vi "Harness_Run All Jitter Tests Reentrancy_Pretest.vi"(10 "Results FilePath":path, 11 "Jitter Test Folder":path) -> ()   [LabVIEW 2009]
panel:
  out "error out":errorcluster
  in  "Run in UI?":bool
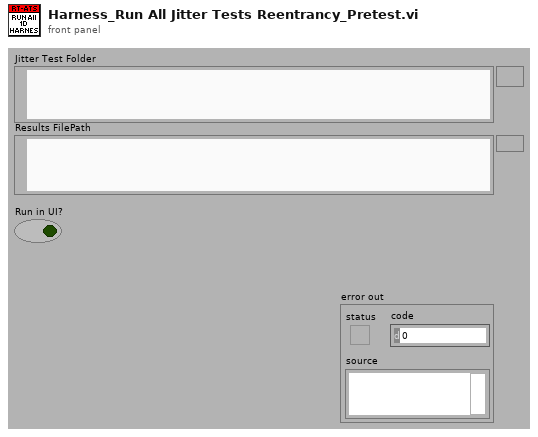
[diagram p1: front panel]
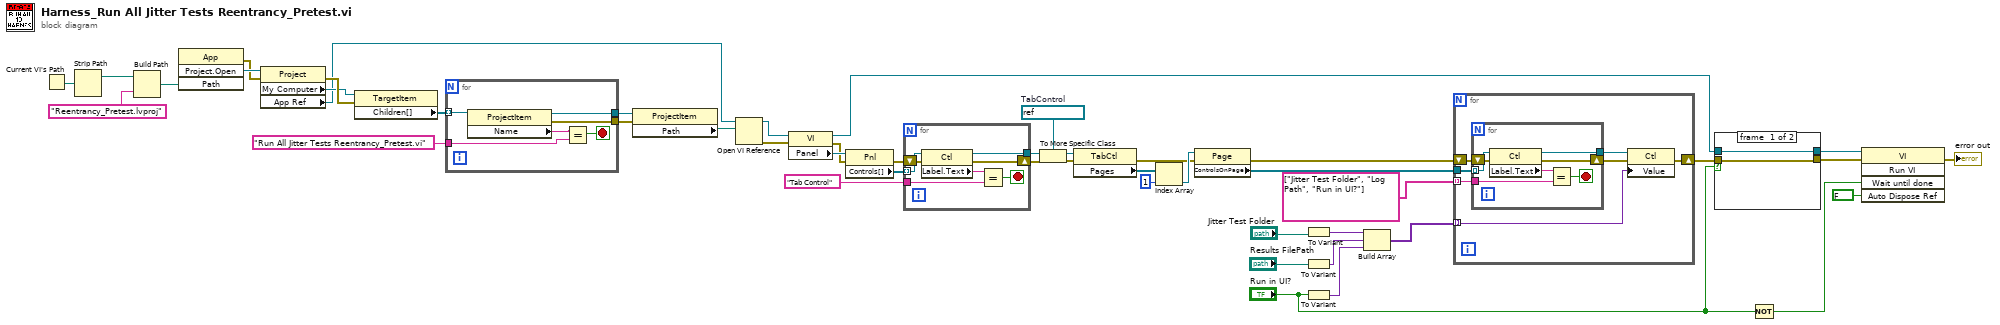
[diagram p0: block diagram]
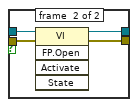
[diagram p2: hidden frame]
diagram:
  w9 = refnum<vi> refnum  # TabControl
  n1 = Current VI's Path() -> (path=w47:path)
  n2 = Strip Path(path=w47) -> (stripped path=w46:path)  [unwired: 1 out]
  n3 = Build Path(base path=w46, name or relative path="Reentrancy_Pretest.lvproj") -> (appended path=w44:path)
  n4 = invoke class="App" method="Project.Open"("Path"=w44) -> (error out=w42:errorcluster, "Project:Open"=w43:refnum<vi>)  [unwired: 3 in, 2 out]
  n5 = property class="Project"(reference=w43, error in=w42) -> (error out=w41:errorcluster, "My Computer"=w35:refnum<vi>, "App Ref"=w34:refnum<vi>)  [unwired: 1 out]
  n6 = property class="TargetItem"(reference=w35, error in=w41) -> ("Children[]"=w40:refnum<vi>[])  [unwired: 2 out]
  n7 = for {
    tunnel: w40 -> [w53] mode=indexing
    tunnel: "Run All Jitter Tests Reentrancy_Pretest.vi" ("name or relative path") -> [w51]
    tunnel: [w49] -> w38
    tunnel: [w48] -> w37
    stop <- w50 stop-if-true
    n8 = property class="ProjectItem"(reference=w53) -> (reference out=w49:refnum<vi>, error out=w48:errorcluster, "Name"=w52:string)  [unwired: 1 in]
    n9 = Equal?(x=w52, y=w51) -> (x = y?=w50:bool)
  }
  n10 = property class="ProjectItem"(reference=w38, error in=w37) -> ("Path"=w36:path)  [unwired: 2 out]
  n11 = Open VI Reference(application reference (local)=w34, vi path=w36) -> (vi reference=w32:refnum<vi>, error out=w33:errorcluster)  [unwired: 4 in]
  n12 = property class="VI"(reference=w32, error in=w33) -> (reference out=w21:refnum<vi>, error out=w30:errorcluster, "Panel"=w31:refnum<vi>)
  n13 = property class="Pnl"(reference=w31, error in=w30) -> (error out=w14:errorcluster, "Controls[]"=w12:refnum<vi>[])  [unwired: 1 out]
  n14 = for {
    tunnel: w12 -> [w59] mode=indexing
    tunnel: "Tab Control" -> [w57]
    tunnel: [w55] -> w11
    shift-right: [w54] -> w10
    shift-left: w14 -> [w60]
    stop <- w56 stop-if-true
    n15 = property class="Ctl"(reference=w59, error in=w60) -> (reference out=w55:refnum<vi>, error out=w54:errorcluster, "Label.Text"=w58:string)
    n16 = Equal?(x=w58, y=w57) -> (x = y?=w56:bool)
  }
  n17 = To More Specific Class(target class=w9, reference=w11, error in=w10) -> (specific class reference=w8:refnum<vi>, error out=w7:errorcluster)
  n18 = property class="TabCtl"(reference=w8, error in=w7) -> (error out=w2:errorcluster, "Pages"=w6:refnum<vi>[])  [unwired: 1 out]
  n19 = Index Array(array=w6, index=1) -> (element=w4:refnum<vi>)
  n20 = property class="Page"(reference=w4, error in=w2) -> (error out=w1:errorcluster, "ControlsOnPage"=w3:refnum<vi>[])  [unwired: 1 out]
  n21 = To Variant(anything="Jitter Test Folder") -> (Variant=w26:variant)
  n22 = To Variant(anything="Results FilePath") -> (Variant=w25:variant)
  n23 = To Variant(anything="Run in UI?") -> (Variant=w24:variant)
  n24 = Build Array(w26, w25, w24) -> (w23:variant[])
  n25 = for {
    tunnel: w3 -> [w67]
    tunnel: string[] ["Jitter Test Folder", "Log Path", "Run in UI?"] -> [w65] mode=indexing
    tunnel: w23 -> [w63] mode=indexing
    shift-right: [w62] -> w22
    shift-left: w1 -> [w66]
    n26 = for {
      tunnel: w67 -> [w73] mode=indexing
      tunnel: w65 -> [w71]
      tunnel: [w69] -> w64
      shift-right: [w68] -> w61
      shift-left: w66 -> [w74]
      stop <- w70 stop-if-true
      n27 = property class="Ctl"(reference=w73, error in=w74) -> (reference out=w69:refnum<vi>, error out=w68:errorcluster, "Label.Text"=w72:string)
      n28 = Equal?(x=w72, y=w71) -> (x = y?=w70:bool)
    }
    n29 = property class="Ctl"(reference=w64, error in=w61, "Value"=w63) -> (error out=w62:errorcluster)  [unwired: 1 out]
  }
  n30 = case shown="True" "Run in UI?" {
    tunnel: w22 -> [w75 w80]
    tunnel: w21 -> [w76 w79]
    tunnel: [w75 w78] -> w20
    tunnel: [w76 w77] -> w19
    frame #0 {
    }
    frame #1 {
      n31 = invoke class="VI" method="FP.Open"(reference=w79, error in=w80) -> (reference out=w77:refnum<vi>, error out=w78:errorcluster)  [unwired: 3 in, 3 out]
    }
  }
  n32 = Not(x="Run in UI?") -> (.not. x?=w17:bool)
  n33 = invoke class="VI" method="Run VI"(reference=w19, error in=w20, "Wait until done"=w17, "Auto Dispose Ref"=FALSE ("Auto Dispose Reference")) -> (error out=→"error out":errorcluster)  [unwired: 1 in, 4 out]
